vi "Read Timer Status.vi"(0 "VISA resource name":refnum<visa-resource-name>, 1 "Unit Address (1)":u8=1 min=1 max=254, 11 "error in (no error)":errorcluster) -> (4 "VISA resource name out":refnum<visa-resource-name>, 6 "Timer Status\n- Decimal":i16(ring) items=["Reset", "Run", "Hold", "End"], 15 "error out":errorcluster)   [LabVIEW 2010, in "Eurotherm 32xx Series.lvlib"]
doc: "This VI returns the current state of the timer"
uses:
  <instrlib>/Eurotherm 32xx Series/Eurotherm 32xx Series.lvlib
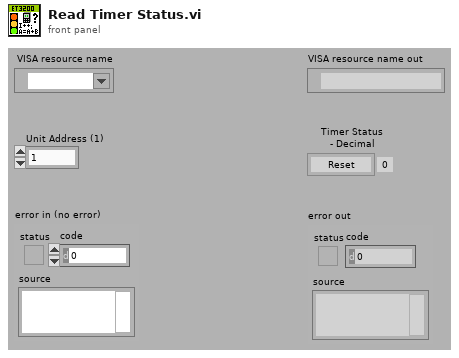
[diagram p1: front panel]
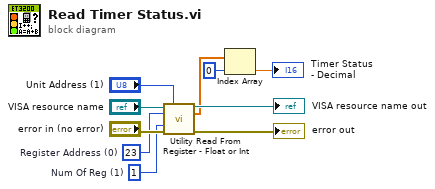
[diagram p0: block diagram]
diagram:
  w2 = u16 23  # Register Address (0)
  w6 = u16 1  # Num Of Reg (1)
  n1 = call <instrlib>:"Utility Read From Register - Float or Int.vi"("VISA resource name"="VISA resource name", "Unit Address (1)"="Unit Address (1)", "Register Address (0)"=w2, "Num Of Reg (1)"=w6, "error in (no error)"="error in (no error)") -> ("VISA resource name out"=→"VISA resource name out":refnum<visa-resource-name>, "Data"=w4:sgl[], "error out"=→"error out":errorcluster)  [unwired: 8 in]
  n2 = Index Array(array=w4, index=0) -> (element=→"Timer Status\n- Decimal":sgl)
